vi "New.vi"(11 "TEMPLATE Msg Output in":refnum<class "TEMPLATE Msg Output.lvclass">) -> (0 "Error out":errorcluster, 3 "TEMPLATE Msg Output out":refnum<class "TEMPLATE Msg Output.lvclass">)   [LabVIEW 2020, in "_Template.lvlib" / "Templates.lvlib" / "TEMPLATE jettl Msg.lvlib" / "TEMPLATE Msg Output.lvclass"]
uses:
  TEMPLATE Msg Output.lvclass
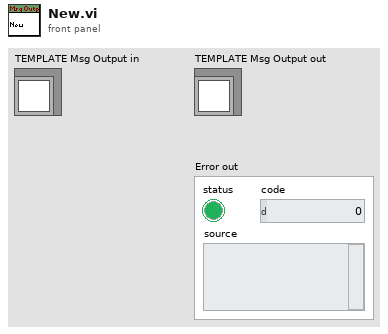
[diagram p1: front panel]
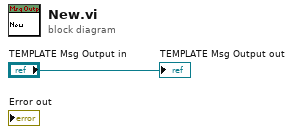
[diagram p0: block diagram]
diagram:
  "TEMPLATE Msg Output out" <- "TEMPLATE Msg Output in"
